vi "Disconnect.vi"(7 "error in (no error)":errorcluster, 10 "Ultimus V in":refnum<class "Ultimus V.lvclass">) -> (0 "error out":errorcluster)   [LabVIEW 2016, in "Ultimus V.lvclass"]
uses:
  Ultimus V.lvclass
  Ultimus V.lvclass/Ultimus V.ctl
  Drivers/EFD Ultimus V/EFD Ultimus V.lvlib
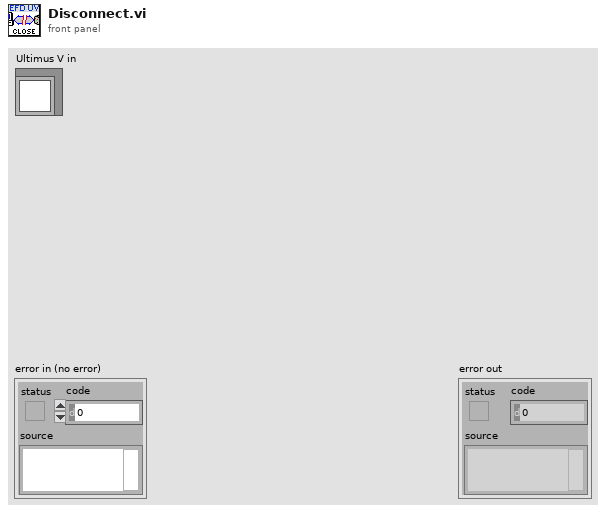
[diagram p1: front panel]
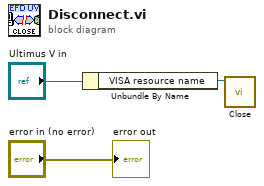
[diagram p0: block diagram]
diagram:
  n1 = Unbundle By Name("Ultimus V in") -> ("VISA resource name"=w2:refnum<visa-resource-name>)
  n2 = call "Close.vi"("VISA resource name"=w2) -> ()  [unwired: 10 in, 1 out]
  "error out" <- "error in (no error)"
